vi "SystemInit.vi"(8 "error in (no error)":errorcluster) -> (0 "error out":errorcluster, 2 "Pound":refnum<class "Pound.lvclass">, 3 "Qbus out":refnum<class "Qbus.lvclass">)   [LabVIEW 2015, in "System.lvlib"]
uses:
  System.lvlib
  <vilib>/addons/Qbus/Qbus.lvclass
  <vilib>/NI/Software Watchdog/Pound/Pound.lvclass
  FileHandler/FileHandler.lvlib
  <vilib>/addons/TimerProcess/TimerProcess.lvlib
  MainController/MainController.lvlib
  ConfigHelper/ConfigHelper.lvlib
  CopyUtility/CopyUtility.lvlib
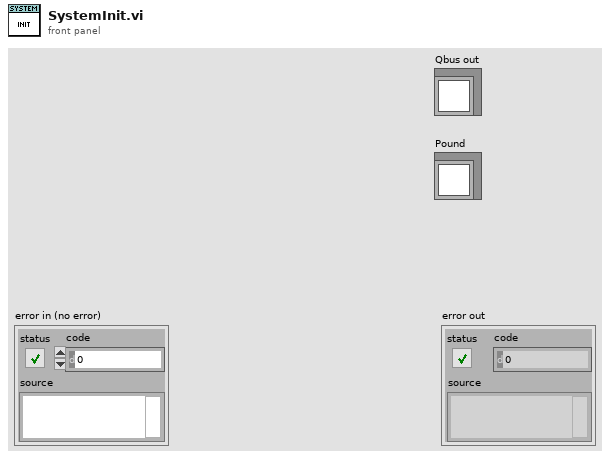
[diagram p1: front panel]
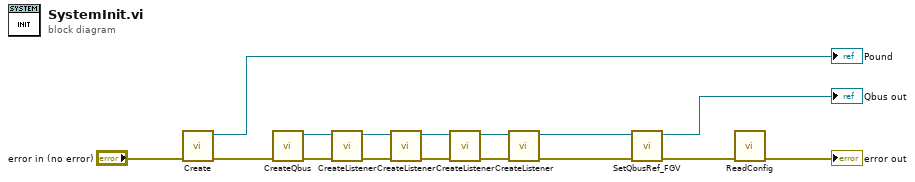
[diagram p0: block diagram]
diagram:
  n1 = call <vilib>:"Create.vi"("error in (no error)"="error in (no error)") -> ("error out"=w12:errorcluster, "Pound"=→"Pound":refnum<class "Pound.lvclass">)  [unwired: 9 in]
  n2 = call <vilib>:"CreateQbus.vi"("error in (no error)"=w12) -> ("error out"=w15:errorcluster, "Qbus"=w16:refnum<class "Qbus.lvclass">)  [unwired: 9 in]
  n3 = call <vilib>:"CreateListener.vi"("error in (no error)"=w15, "qbus in"=w16) -> ("error out"=w13:errorcluster, "qbus out"=w14:refnum<class "Qbus.lvclass">)  [unwired: 8 in]
  n4 = call <vilib>:"CreateListener.vi"("error in (no error)"=w13, "qbus in"=w14) -> ("error out"=w8:errorcluster, "qbus out"=w9:refnum<class "Qbus.lvclass">)  [unwired: 8 in]
  n5 = call <vilib>:"CreateListener.vi"("error in (no error)"=w8, "qbus in"=w9) -> ("error out"=w6:errorcluster, "qbus out"=w7:refnum<class "Qbus.lvclass">)  [unwired: 8 in]
  n6 = call <vilib>:"CreateListener.vi"("error in (no error)"=w6, "qbus in"=w7) -> ("error out"=w1:errorcluster, "qbus out"=w2:refnum<class "Qbus.lvclass">)  [unwired: 8 in]
  n7 = call <vilib>:"SetQbusRef_FGV.vi"("error in (no error)"=w1, "Qbus in"=w2) -> ("error out"=w4:errorcluster, "Qbus out"=→"Qbus out":refnum<class "Qbus.lvclass">)  [unwired: 8 in]
  n8 = call "ReadConfig.vi"("error in (no error)"=w4) -> ("error out"=→"error out":errorcluster)  [unwired: 9 in, 1 out]
